vi "TransactionInDb.vi"() -> ()   [LabVIEW 2019]
uses:
  <vilib>/addons/database/Auxilliary.llb/DB Tools Transaction.ctl
  <vilib>/addons/database/Auxilliary.llb/DB Tools Column Info.ctl
  <vilib>/addons/database/Auxilliary.llb/DB Tools DataTypes.ctl
  <vilib>/addons/database/Connection.llb/DB Tools Open Connec (String).vi
  <vilib>/addons/database/Connection.llb/Conn Transaction.vi
  <vilib>/addons/database/NI_Database_API.lvlib
panel:
  in  "Enter Your Table Name Here":string
  in  "Provide Your ODBC Server Name":string
  # "Integity of the database is very important because Multiple users can have access for the same database"
  # "And they can Manipulate the same data many time In this case Transactions come into existance which assured that"
  # "the ACID rule of the databse will be maintained in any scenerio .  Basically transactions assured  that either whole recordset will be"
  # "updated into Db or no changes will be inserted .. We will bind many opreations inside the same Transaction . Transactions"
  # "contains two thing end transaction VI and Stop transactions VI.`"
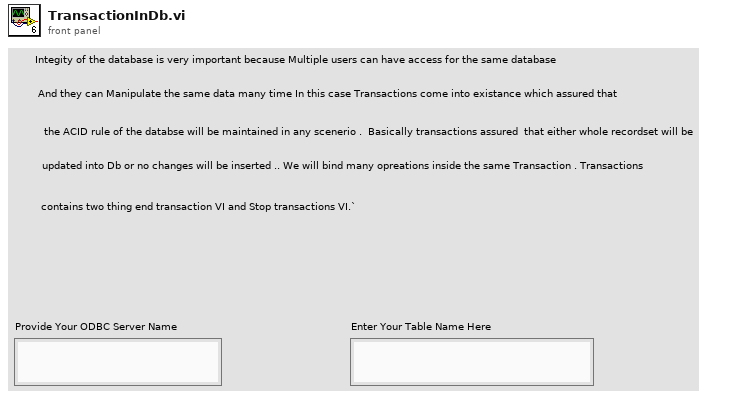
[diagram p1: front panel]
types:
  T1 = typedef "NI_Database_API.lvlib/DB Tools Transaction.ctl" = enum16{"begin", "commit", "rollback"}
  T2 = typedef "NI_Database_API.lvlib/DB Tools Column Info.ctl" = cluster{"column name":string, "data type":T3, "size":i32, "allow null?":bool}
  T3 = typedef "NI_Database_API.lvlib/DB Tools DataTypes.ctl" = enum16{"String", "Long (I32)", "Single (SGL)", "Double (DBL)", "Date/Time", "Binary"}
  T4 = typedef "NI_Database_API.lvlib/Conn ObjectReference.ctl" = refnum<k1>
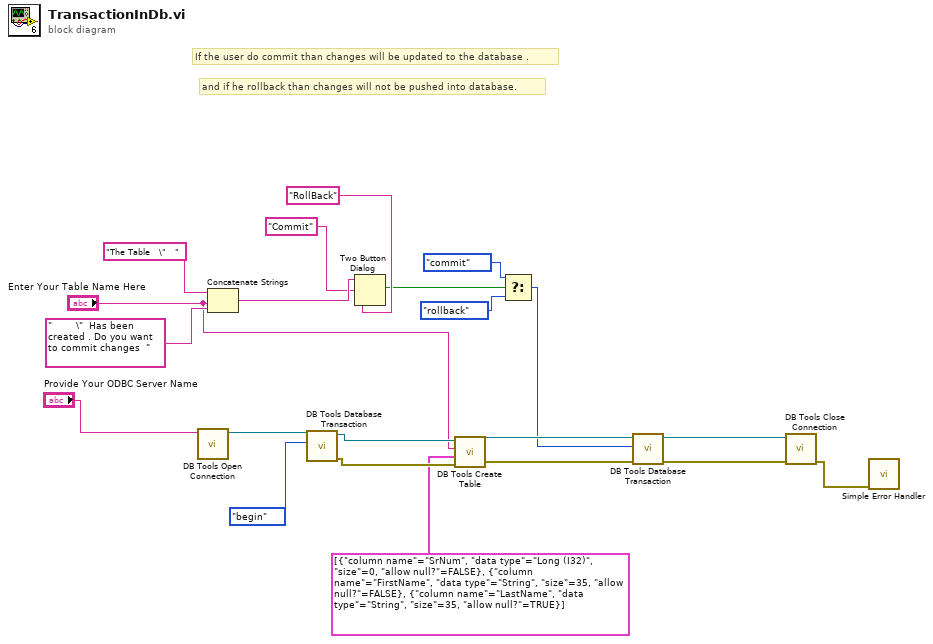
[diagram p0: block diagram]
diagram:
  # "and if he rollback than changes will not be pushed into database."
  # "If the user do commit than changes will be updated to the database ."
  n1 = call-poly <vilib>:"DB Tools Open Connection.vi"("connection information"="Provide Your ODBC Server Name") -> ("connection reference"=w20:T4)  [unwired: 7 in, 1 out]
  n2 = Concatenate Strings("The Table   \"   " ("string"), "Enter Your Table Name Here", "        \"  Has been created . Do you want to commit changes  " ("string")) -> (w14:string)
  n3 = call-poly <vilib>:"DB Tools Database Transaction.vi"("operation (begin)"=DB_Tools_Transaction."begin", "connection reference"=w20) -> ("error out"=w17:errorcluster, "connection reference out"=w18:T4)  [unwired: 4 in]
  n4 = Two Button Dialog(message=w14, 1:"RollBack" ("F button name (\"Cancel\")"), 2:"Commit" ("T button name (\"OK\")")) -> (T button?=w11:bool)
  n5 = call <vilib>:"DB Tools Create Table.vi"("error in (no error)"=w17, "column information"=T2[] [{"column name"="SrNum", "data type"=enum."Long (I32)", "size"=0, "allow null?"=FALSE}, {"column name"="FirstName", "data type"=enum."String", "size"=35, "allow null?"=FALSE}, {"column name"="LastName", "data type"=enum."String", "size"=35, "allow null?"=TRUE}], "table"="Enter Your Table Name Here", "connection reference"=w18) -> ("error out"=w7:errorcluster, "connection reference out"=w8:T4)  [unwired: 4 in]
  n6 = Select(t=DB_Tools_Transaction."commit" ("operation (begin)"), s=w11, f=DB_Tools_Transaction."rollback" ("operation (begin)")) -> (s? t:f=w6:T1)
  n7 = call-poly <vilib>:"DB Tools Database Transaction.vi"("error in (no error)"=w7, "operation (begin)"=w6, "connection reference"=w8) -> ("error out"=w2:errorcluster, "connection reference out"=w3:T4)  [unwired: 3 in]
  n8 = call <vilib>:"DB Tools Close Connection.vi"("error in (no error)"=w2, "connection reference"=w3) -> ("error out"=w1:errorcluster)  [unwired: 5 in]
  n9 = call <vilib>:"Simple Error Handler.vi"("error in (no error)"=w1) -> ()  [unwired: 4 in, 5 out]
